vi "UserConsole_Timing.vi"() -> (3 "Elapsed?":bool)   [LabVIEW 2013, in "UserConsole.lvlib"]
uses:
  UserConsole.lvlib
panel:
  in  "ElapsedTime(X)":dbl
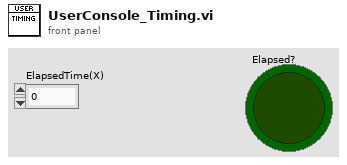
[diagram p1: front panel]
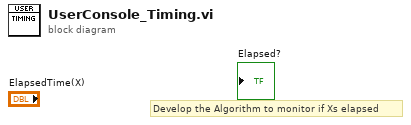
[diagram p0: block diagram]
diagram:
  # "Develop the Algorithm to monitor if Xs elapsed"
